vi "Get VI Window Title.vi"(2 "error in (no error)":errorcluster, 3 "VI Name":string) -> (0 "error out":errorcluster, 1 "Window Title":string)   [LabVIEW 2017]
doc: "Gets the Windows title bar title for the specified VI. The specified VI must already be in memory."
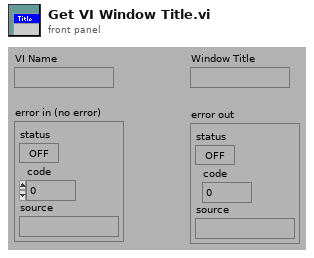
[diagram p1: front panel]
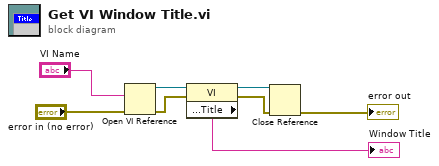
[diagram p0: block diagram]
diagram:
  n1 = Open VI Reference(vi path="VI Name", error in (no error)="error in (no error)") -> (vi reference=w4:refnum<vi>, error out=w5:errorcluster)  [unwired: 4 in]
  n2 = property class="VI"(reference=w4, error in=w5) -> (reference out=w6:refnum<vi>, error out=w7:errorcluster, "Front Panel Window:Title"=→"Window Title":string)
  n3 = Close Reference(reference=w6, error in (no error)=w7) -> (error out=→"error out":errorcluster)
